vi "Scaling.vi"(1 "Measured Voltage":dbl, 2 "Reference R":dbl) -> (0 "Thermistor Res":dbl)   [LabVIEW 2022 SP3]
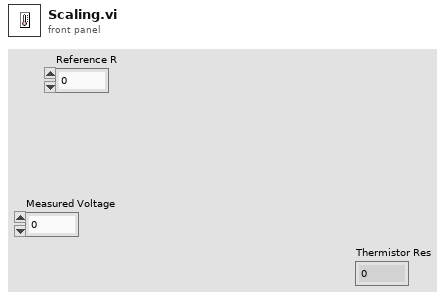
[diagram p1: front panel]
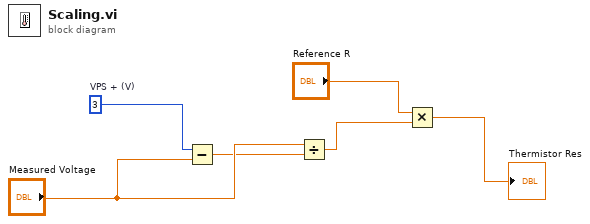
[diagram p0: block diagram]
diagram:
  w6 = 3  # VPS + (V)
  n1 = Subtract(x=w6, y="Measured Voltage") -> (x-y=w4:dbl)
  n2 = Divide(x="Measured Voltage", y=w4) -> (x/y=w2:dbl)
  n3 = Multiply(x="Reference R", y=w2) -> (x*y=→"Thermistor Res":dbl)
